vi "InitModuleTypes.vi"(8 "ErrorArray In":errorcluster[](array[cluster]), 11 "refnum":T1) -> (0 "ErrorArray Out":errorcluster[](array[cluster]))   [LabVIEW 2014, in "Framework.lvlib"]
uses:
  Framework.lvlib
  <vilib>/Utility/config.llb/Config Data RefNum.ctl
  <vilib>/Utility/config.llb/Read Key (String).vi
  <vilib>/Utility/config.llb/NI_LVConfig.lvlib
  <userlib>/NIST/NISTErrorLib/NISTErrorLib.lvlib
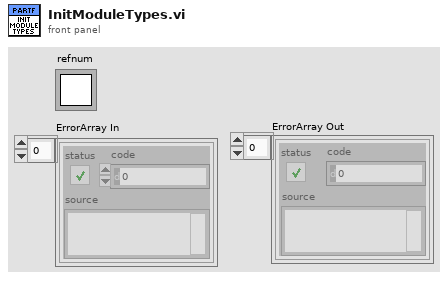
[diagram p1: front panel]
types:
  T1 = typedef "NI_LVConfig.lvlib/Config Data RefNum.ctl" = refnum<k1>
  T2 = typedef "Framework.lvlib/clFrontPanelControlRefs.ctl" = cluster{"TestFilePathRef":refnum<vi>, "BusNumberRef":refnum<vi>, "NumberOfBusesRef":refnum<vi>, "EvtTypeRef":refnum<vi>, "EvtParamsRef":refnum<vi>, "EvtConfigRef":refnum<vi>, "StartTimeRef":refnum<vi>, "EndTimeRef":refnum<vi>, "PmuImpairTypeRef":refnum<vi>, "PmuImpairParamsRef":refnum<vi>, "NetImpairParamsRef":refnum<vi>, "FlagImpairTypeRef":refnum<vi>, "FlagImpairParamsRef":refnum<vi>, "NetImpairTypeRef":refnum<vi>, "OutputFileType":refnum<vi>, "PmuImpairConfigRef":refnum<vi>, "AppTypeRef":refnum<vi>, "ScriptPathRef":refnum<vi>, "ShowPanels?":refnum<vi>}
  T3 = typedef "LVStringsAndValuesArrayTypeDef_U16.ctl" = cluster{"String":string, "Value":u16}[]
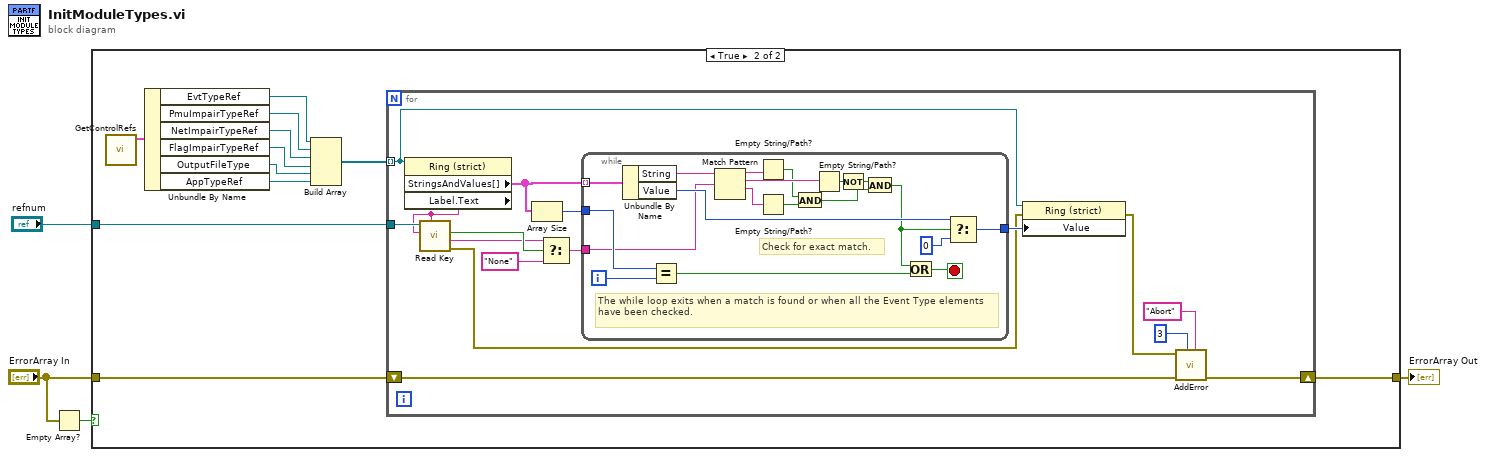
[diagram p0: block diagram]
diagram:
  n1 = Empty Array?(array="ErrorArray In") -> (empty?=w4:bool)
  n2 = case shown="True" w4 {
    tunnel: "ErrorArray In" -> [w5 w7]
    tunnel: [w5 w6] -> w2
    tunnel: "refnum" -> [_ w8]
    frame False {
    }
    frame True {
      n3 = call "GetControlRefs.vi"() -> ("clControlRefs Out"=w10:T2)  [unwired: 11 in]
      n4 = Unbundle By Name(w10) -> ("EvtTypeRef"=w16:refnum<vi>, "PmuImpairTypeRef"=w15:refnum<vi>, "NetImpairTypeRef"=w14:refnum<vi>, "FlagImpairTypeRef"=w13:refnum<vi>, "OutputFileType"=w12:refnum<vi>, "AppTypeRef"=w11:refnum<vi>)
      n5 = Build Array(w16, w15, w14, w13, w12, w11) -> (w9:refnum<vi>[])
      n6 = for {
        tunnel: w9 -> [w30] mode=indexing
        tunnel: w8 -> [w32]
        shift-right: [w18] -> w6
        shift-left: w7 -> [w19]
        n7 = property class="Ring (strict)"(reference=w30) -> ("StringsAndValues[]"=w29:T3, "Label.Text"=w17:string)  [unwired: 1 in, 2 out]
        n8 = call-poly <vilib>:"Read Key.vi"("section"=w17, "key"=w17, "refnum"=w32) -> ("error out"=w23:errorcluster, "value"=w25:string, "found?"=w26:bool)  [unwired: 5 in, 1 out]
        n9 = Array Size(array=w29) -> (size(s)=w28:i32)
        n10 = Select(t=w25, s=w26, f="None" ("regular expression")) -> (s? t:f=w24:string)
        n11 = while {
          tunnel: w29 -> [w39] mode=indexing
          tunnel: [w35] -> w31
          tunnel: w28 -> [w34]
          tunnel: w24 -> [w33]
          i -> [w42]
          stop <- w41 stop-if-true
          # "The while loop exits when a match is found or when all the Event Type elements have been checked."
          # "Check for exact match."
          n12 = Unbundle By Name(w39) -> ("String"=w51:string, "Value"=w38:u16)
          n13 = Equal?(x=w34, y=w42) -> (x = y?=w40:bool)
          n14 = Match Pattern(string=w51, regular expression=w33) -> (before substring=w48:string, match substring=w50:string, after substring=w47:string)  [unwired: 1 in, 1 out]
          n15 = Empty String/Path?(string/path=w48) -> (empty?=w45:bool)
          n16 = Empty String/Path?(string/path=w47) -> (empty?=w46:bool)
          n17 = And(x=w45, y=w46) -> (x .and. y?=w44:bool)
          n18 = Empty String/Path?(string/path=w50) -> (empty?=w49:bool)
          n19 = Not(x=w49) -> (.not. x?=w43:bool)
          n20 = And(x=w43, y=w44) -> (x .and. y?=w36:bool)
          n21 = Or(x=w36, y=w40) -> (x .or. y?=w41:bool)
          n22 = Select(t=w38, s=w36, f=u16 0) -> (s? t:f=w35:u16)
        }
        n23 = property class="Ring (strict)"(reference=w30, error in=w23, "Value"=w31) -> (error out=w22:errorcluster)  [unwired: 1 out]
        n24 = call <userlib>:"AddError.vi"("Severity"="Abort", "Priority"=u8 3, "ErrorArray"=w19, "error in (no error)"=w22) -> ("ErrorArray"=w18:errorcluster[])  [unwired: 6 in, 1 out]
      }
    }
  }
  "ErrorArray Out" <- w2
